vi "Read (I16).vi"(0 "disk streaming in":refnum<class "Disk Streaming.lvclass">, 3 "empty elements remaining":u32, 5 "error in (no error)":errorcluster) -> (13 "finished":bool, 14 "disk streaming out":refnum<class "Disk Streaming.lvclass">, 15 "sample data":i16[](array[numeric]), 18 "number of pending reads":u32, 19 "error out":errorcluster)   [LabVIEW 2021, in "Disk Streaming.lvclass"]
doc: "Reads data from a file in the streaming process controlled by a disk streaming instance and generates status information. For more information about the disk streaming instance refer to the <B>Open.vi</B> context help.\n\nUse this VI when streaming from disk using the TDMS Advanced Synchronous I/O functions or the TDMS Advanced Asynchronous I/O functions (the disk streaming instance was created by the <B>Open.vi</B> with the <B>disk read (F) / write (T)</B> input set to false and the <B>I/O mode</B> input set to \"Synchronous\" or \"Asynchronous\"). The streaming process requires the execution of the following sequence in a loop:\n1. Call this VI to read the data to transfer in the current iteration. The <B>finished</B> output of this VI signals whether this transfer completes the streaming.\n2. Call the Write FIFO method on the Host to Target FIFO transferring the data to the FPGA Target to write the data to the host DMA buffer. Use the array returned by this VI on the \"Data\" input of the FIFO method.\n\nInputs:\n\n<B>disk streaming in</B>: Disk streaming instance input.\n\n<B>empty elements remaining</B>: Set this input to the number of additional empty elements remaining in the host DMA buffer that are available for writing. This input is used only in the calculation of the Host DMA buffer utilization status. Wire the \"Empty Elements Remaining\" output of the FIFO method writing the Host to Target FIFO buffer to this input.\n\nOutputs:\n\n<B>disk streaming out</B>: Disk streaming instance output. Pass this output to the other Disk Streaming VIs to perform the streaming.\n\n<B>sample data</B>: Array of I16s read from the file. Wire this output to the \"Data\" input of the FIFO method writing the Host to Target FIFO buffer.\n\n<B>number of pending reads</B>: The number of asynchronous reads that are currently running in the background. Use the <B>Get Status.vi</B> to obtain additional status information.\n\n<B>finished</B>: Indicates whether the streaming is finished."
uses:
  Disk Streaming.lvclass
  Disk Streaming.lvclass/Disk Streaming.ctl
  <vilib>/Utility/error.llb/Error Cluster From Error Code.vi
  <vilib>/ErrorRing/Error Ring.xnode
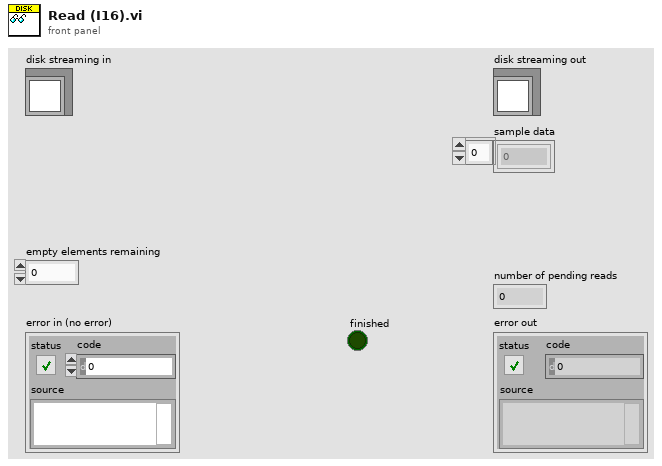
[diagram p1: front panel]
types:
  T1 = typedef "Disk Streaming.lvclass/Data.ctl" = cluster{"tdms file":refnum<k34>, "group name":string, "channel name":string, "max operations":u32, "timeout (s)":dbl, "data type size (bytes)":u64, "writing":bool, "I/O mode":T2, "# of blocks":u32, "block size divisor (bytes)":u32, "file position (elements)":u64, "file size (elements)":i64, "file size (samples)":i64, "block size (elements)":u64, "block size (samples)":u64, "quantum size (elements)":u64, "quantum size (samples)":u64, "samples remaining":i64, "elements transferred":u64, "finished":bool, "preview size":i32, "preview quantum size (elements)":u64, "preview quantum size (samples)":u64, "DMA buffer size (elements)":u32, "pending block sizes (bytes)":u64[]}
  T2 = typedef "Disk Streaming.lvclass/IO mode.ctl" = enum16{"Synchronous", "Asynchronous", "Data Reference"}
  T3 = typedef "Disk Streaming.lvclass/Status.ctl" = cluster{"finished":bool, "Host DMA buffer size (bytes)":u64, "Host DMA buffer utilization (bytes)":u64, "Disk maximum async operations":u32, "Disk pending async operations":u32, "preview data":i16[]}
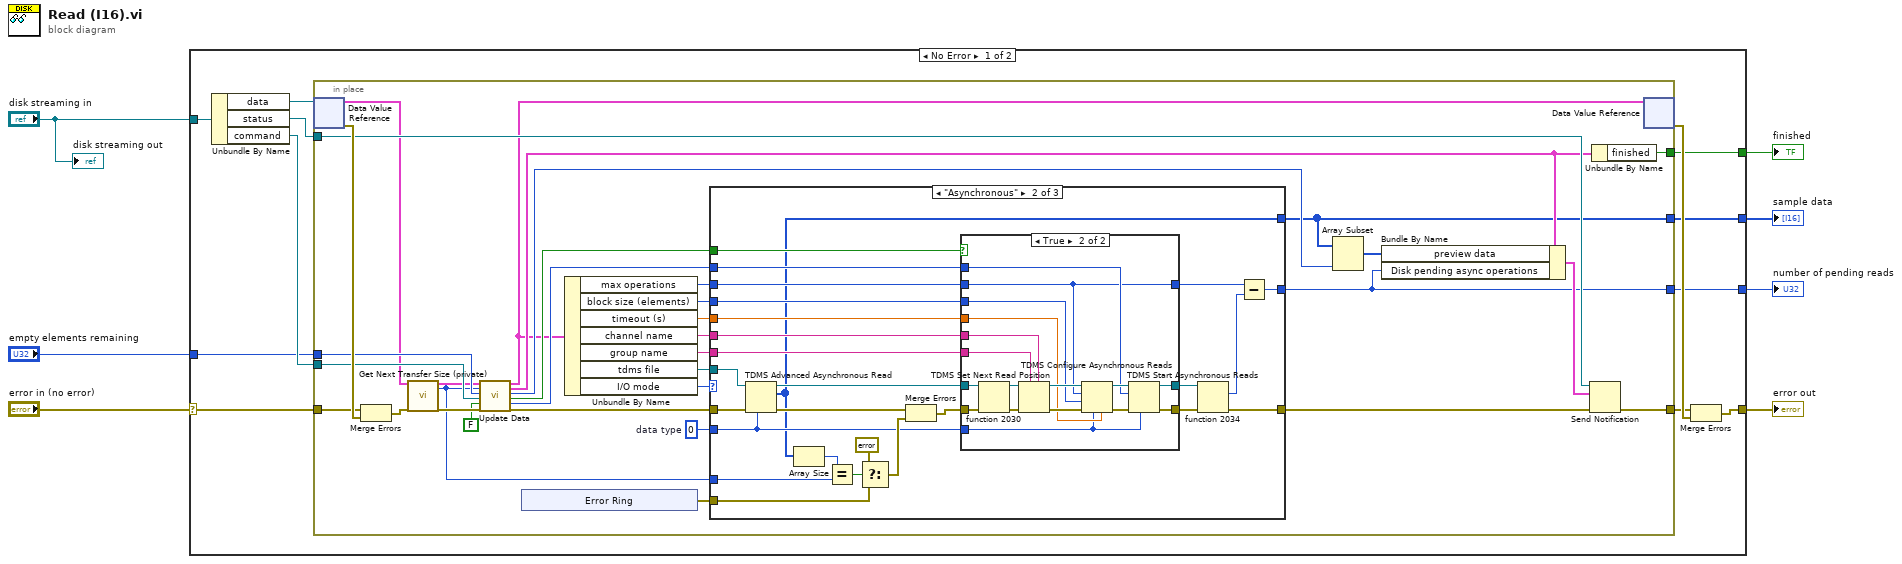
[diagram p0: block diagram]
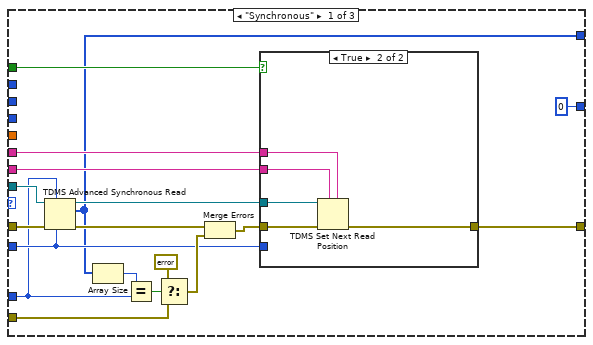
[diagram p2: hidden frame]
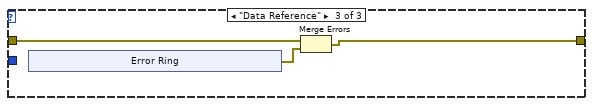
[diagram p5: hidden frame]
diagram:
  n1 = case shown="No Error" "error in (no error)" {
    selector: "error in (no error)" -> [w17 w136]
    tunnel: [w16 w136] -> w6
    tunnel: [w14 _] -> w5
    tunnel: "empty elements remaining" -> [w11 _]
    tunnel: "disk streaming in" -> [w13 _]
    tunnel: [w9 _] -> w2
    tunnel: [w8 _] -> w1
    frame No Error {
      n2 = Unbundle By Name(w13) -> ("data"=w12:refnum<data-value>, "status"=w10:refnum<notifier>, "command"=w19:refnum<notifier>)
      n3 = in-place {
        in-place-border: w17 -> [w47]
        in-place-border: [w42] -> w15
        in-place-border: [w34] -> w14
        in-place-border: w19 -> [w44]
        in-place-border: w11 -> [w45]
        in-place-border: w10 -> [w48]
        in-place-border: [w41] -> w9
        in-place-border: [w22] -> w8
        w30 = i16 0  # data type
        n4 = in-place-dvr #1(w12) -> (w37:T1, w49:errorcluster)
        n5 = Merge Errors(w47, w49) -> (w38:errorcluster)
        n6 = call "Get Next Transfer Size (private).vi"("data in"=w37, "error in (no error)"=w38) -> ("data out"=w36:T1, "elements to transfer"=w27:u32, "error out"=w51:errorcluster)  [unwired: 15 in]
        n7 = call "Update Data.vi"("data in"=w36, "block size (elements)"=w27, "(empty) elements remaining"=w45, "command"=w44, "writing?"=FALSE, "error in (no error)"=w51) -> ("data out"=w23:T1, "status"=w39:T3, "preview size (elements)"=w52:i32, "reopen file"=w25:bool, "reopen total count (elements)"=w24:i64, "error out"=w50:errorcluster)  [unwired: 8 in]
        n8 = xnode "Error Ring"() -> ("error out"=w20:errorcluster)
        n9 = Unbundle By Name(w23) -> ("max operations"=w33:u32, "block size (elements)"=w32:u64, "timeout (s)"=w31:dbl, "channel name"=w29:string, "group name"=w28:string, "tdms file"=w35:refnum<k34>, "I/O mode"=w21:T2)
        n10 = case shown="\"Asynchronous\"" w21 {
          tunnel: w50 -> [w73 w105 w130]
          tunnel: w35 -> [w72 w104 _]
          tunnel: [u32 0 w102 _] -> w34
          tunnel: w33 -> [_ w101 _]
          tunnel: w32 -> [_ w97 _]
          tunnel: w31 -> [_ w96 _]
          tunnel: w30 -> [w70 w95 _]
          tunnel: w29 -> [w69 w94 _]
          tunnel: w28 -> [w68 w93 _]
          tunnel: w27 -> [w60 w91 _]
          tunnel: [w59 w86 w129] -> w26
          tunnel: w25 -> [w63 w85 _]
          tunnel: w24 -> [_ w84 _]
          tunnel: [w62 w83 _] -> w22
          tunnel: w20 -> [w61 w82 _]
          frame "Synchronous" {
            n11 = TDMS Advanced Synchronous Read(6:w70, 7:w60, 8:w73, 11:w72) -> (0:w75:errorcluster, 2:w62:i16[], 3:w71:refnum<k34>)  [unwired: 1 out]
            n12 = Array Size(array=w62) -> (size(s)=w67:i32)
            n13 = Equal?(x=w67, y=w60) -> (x = y?=w66:bool)
            n14 = Select(t=errorcluster {"status"=FALSE, "code"=0, "source"=""}, s=w66, f=w61) -> (s? t:f=w74:errorcluster)
            n15 = Merge Errors(w75, w74) -> (w64:errorcluster)
            n16 = case shown="True" w63 {
              tunnel: [w76 w77] -> w59
              tunnel: w71 -> [_ w78]
              tunnel: w70 -> [_ _]
              tunnel: w69 -> [_ w81]
              tunnel: w68 -> [_ w80]
              tunnel: w64 -> [w76 w79]
              frame False {
              }
              frame True {
                n17 = TDMS Set Next Read Position(5:w81, 7:w80, 8:w79, 11:w78) -> (0:w77:errorcluster)  [unwired: 2 in, 1 out]
              }
            }
          }
          frame "Asynchronous" {
            n18 = TDMS Advanced Asynchronous Read(6:w95, 8:w105, 11:w104) -> (0:w107:errorcluster, 2:w83:i16[], 3:w98:refnum<k34>)  [unwired: 1 out]
            n19 = Array Size(array=w83) -> (size(s)=w92:i32)
            n20 = Equal?(x=w92, y=w91) -> (x = y?=w90:bool)
            n21 = Select(t=errorcluster {"status"=FALSE, "code"=0, "source"=""}, s=w90, f=w82) -> (s? t:f=w106:errorcluster)
            n22 = Merge Errors(w107, w106) -> (w88:errorcluster)
            n23 = case shown="True" w85 {
              tunnel: w101 -> [w110 w111]
              tunnel: [w108 w121] -> w100
              tunnel: [w109 w120] -> w99
              tunnel: w98 -> [w109 w119]
              tunnel: w97 -> [_ w118]
              tunnel: w96 -> [_ w117]
              tunnel: w95 -> [_ w116]
              tunnel: w84 -> [_ w115]
              tunnel: w94 -> [_ w114]
              tunnel: w93 -> [_ w113]
              tunnel: w88 -> [w108 w112]
              tunnel: [w110 w111] -> w87
              frame False {
              }
              frame True {
                n24 = fn#2030(8:w112, 11:w119) -> (0:w125:errorcluster, 3:w124:refnum<k34>)
                n25 = TDMS Set Next Read Position(5:w114, 7:w113, 8:w125, 11:w124) -> (0:w122:errorcluster, 3:w123:refnum<k34>)  [unwired: 2 in]
                n26 = TDMS Configure Asynchronous Reads(4:w117, 6:w116, 8:w122, 9:w118, 10:w111, 11:w123) -> (0:w127:errorcluster, 3:w126:refnum<k34>)
                n27 = TDMS Start Asynchronous Reads(6:w116, 8:w127, 10:w115, 11:w126) -> (0:w121:errorcluster, 3:w120:refnum<k34>)
              }
            }
            n28 = fn#2034(8:w100, 11:w99) -> (0:w86:errorcluster, 2:w103:u32)  [unwired: 2 out]
            n29 = Subtract(x=w87, y=w103) -> (x-y=w102:u32)
          }
          frame "Data Reference" {
            n30 = xnode "Error Ring"() -> ("error out"=w128:errorcluster)
            n31 = Merge Errors(w130, w128) -> (w129:errorcluster)
          }
        }
        n32 = Array Subset(array=w22, length=w52) -> (w40:i16[])  [unwired: 1 in]
        n33 = Bundle By Name(cluster=w39, "preview data"=w40, "Disk pending async operations"=w34) -> (w46:T3)
        n34 = Send Notification(notification=w46, notifier=w48, error in (no error)=w26) -> (error out=w42:errorcluster)  [unwired: 1 out]
        n35 = Unbundle By Name(w39) -> ("finished"=w41:bool)
        n36 = in-place-dvr #1(w23) -> (w18:errorcluster)  [unwired: 1 out]
      }
      n37 = Merge Errors(w15, w18) -> (w16:errorcluster)
    }
    frame Error {
    }
  }
  "error out" <- w6
  "sample data" <- w1
  "number of pending reads" <- w5
  "finished" <- w2
  "disk streaming out" <- "disk streaming in"
